vi "红绿灯.vi"() -> ()   [LabVIEW 2020]
panel:
  in  "布尔":bool caption="白天/黑夜模式"
  out "簇 十位  2":T1
  out "簇 个位 2":T1
  out "簇 十位":T1
  out "簇 个位":T1
  in  "停止":bool
  out "Elapsed Time (s)":dbl caption="已用时间(s)"
  out "南北绿[5]":bool
  out "南北黄[4]":bool
  out "南北红[3]":bool
  out "东西绿[2]":bool
  out "东西黄[1]":bool
  out "东西红[0]":bool
  # "北"
  # "西"
  # "东"
  # "南"
  # "白天"
  # "黑夜"
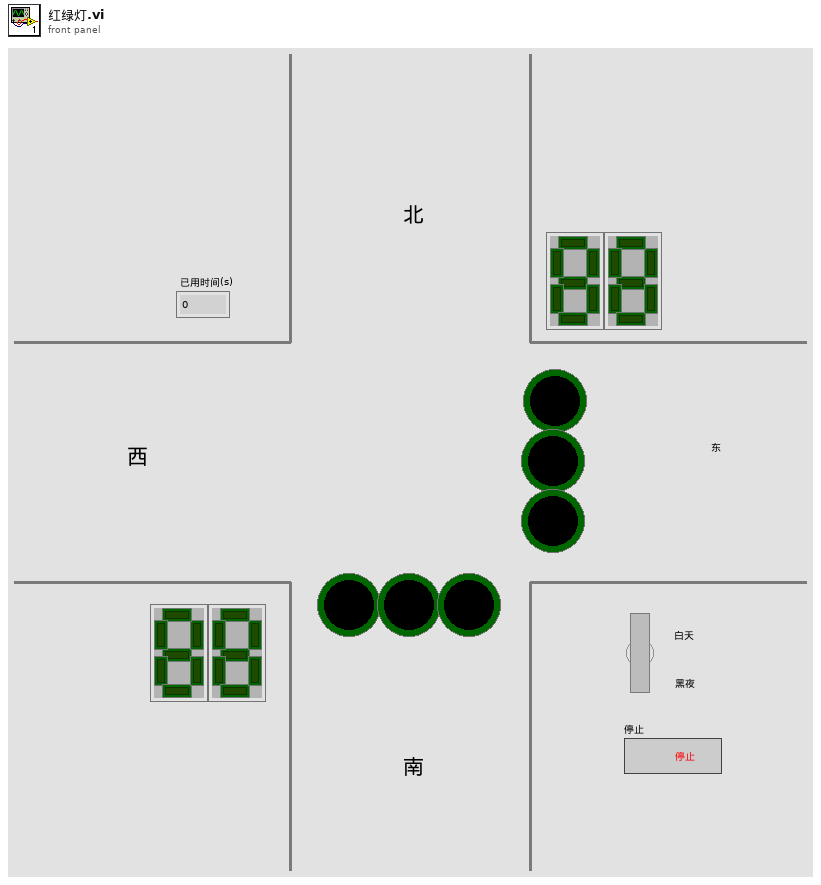
[diagram p1: front panel]
types:
  T1 = cluster{"布尔":bool, "布尔 2":bool, "布尔 3":bool, "布尔 4":bool, "布尔 5":bool, "布尔 6":bool, "布尔 7":bool}
  T2 = cluster{"布尔[0]":bool, "布尔[1]":bool, "布尔[2]":bool, "布尔[3]":bool, "布尔[4]":bool, "布尔[5]":bool}
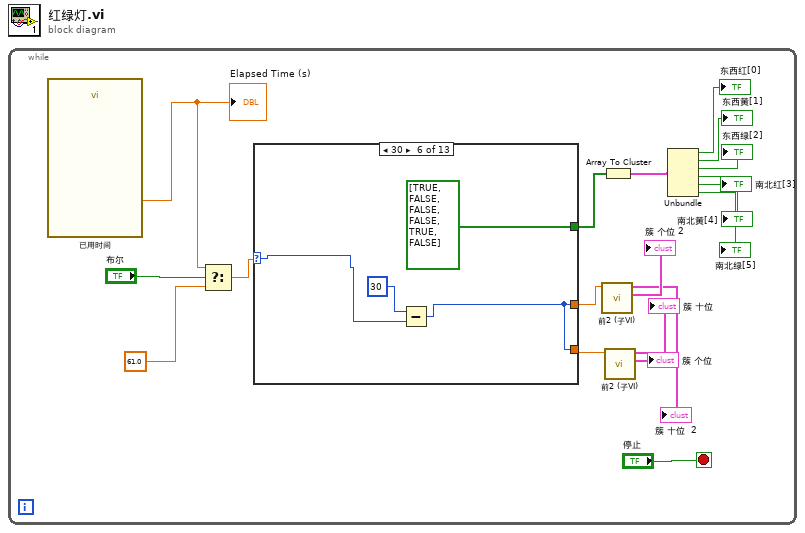
[diagram p0: block diagram]
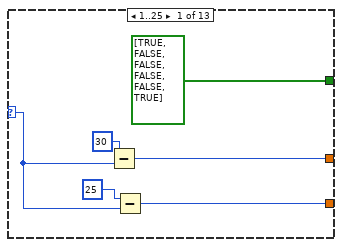
[diagram p2: hidden frame]
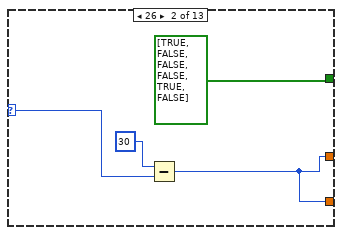
[diagram p3: hidden frame]
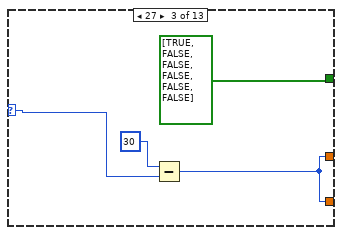
[diagram p4: hidden frame]
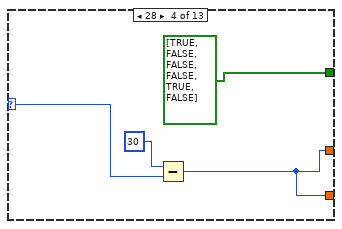
[diagram p5: hidden frame]
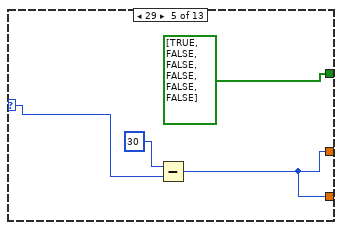
[diagram p6: hidden frame]
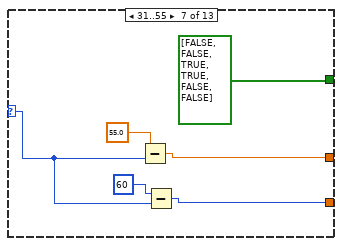
[diagram p7: hidden frame]
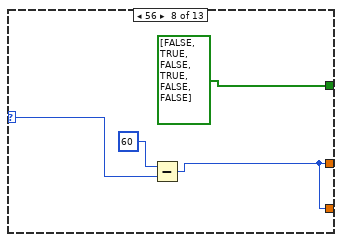
[diagram p8: hidden frame]
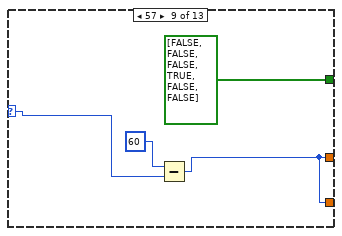
[diagram p9: hidden frame]
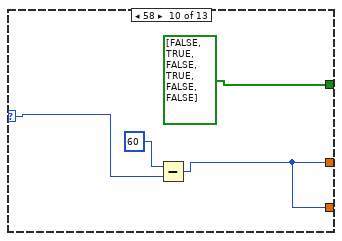
[diagram p10: hidden frame]
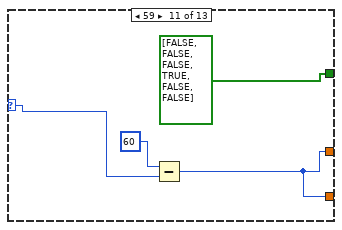
[diagram p11: hidden frame]
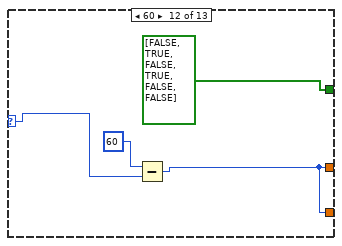
[diagram p12: hidden frame]
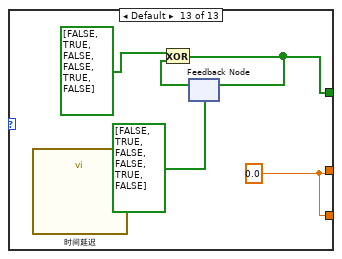
[diagram p13: hidden frame]
diagram:
  n1 = while {
    stop <- "停止" stop-if-true
    n2 = call "已用时间"() -> ("Elapsed Time (s)"=w11:dbl)  [unwired: 12 in, 7 out]
    "Elapsed Time (s)" <- w11
    n3 = Select(t=w11, s="布尔", f=61.0) -> (s? t:f=w8:dbl)
    n4 = case shown="30" w8 {
      selector: w8 -> [w20 w27 w32 w35 w39 w43 w48 w53 w57 w61 w65 w69 _]
      tunnel: [bool[] [TRUE, FALSE, FALSE, FALSE, FALSE, TRUE] ("布尔") bool[] [TRUE, FALSE, FALSE, FALSE, TRUE, FALSE] ("布尔") bool[] [TRUE, FALSE, FALSE, FALSE, FALSE, FALSE] ("布尔") bool[] [TRUE, FALSE, FALSE, FALSE, TRUE, FALSE] ("布尔") bool[] [TRUE, FALSE, FALSE, FALSE, FALSE, FALSE] ("布尔") bool[] [TRUE, FALSE, FALSE, FALSE, TRUE, FALSE] ("布尔") bool[] [FALSE, FALSE, TRUE, TRUE, FALSE, FALSE] ("布尔") bool[] [FALSE, TRUE, FALSE, TRUE, FALSE, FALSE] ("布尔") bool[] [FALSE, FALSE, FALSE, TRUE, FALSE, FALSE] ("布尔") bool[] [FALSE, TRUE, FALSE, TRUE, FALSE, FALSE] ("布尔") bool[] [FALSE, FALSE, FALSE, TRUE, FALSE, FALSE] ("布尔") bool[] [FALSE, TRUE, FALSE, TRUE, FALSE, FALSE] ("布尔") w75] -> w19
      tunnel: [w24 w26 w31 w34 w38 w42 w47 w52 w56 w60 w64 w68 w72] -> w6
      tunnel: [w23 w26 w31 w34 w38 w42 w46 w52 w56 w60 w64 w68 w72] -> w5
      frame 1..25 {
        n5 = Subtract(x=30, y=w20) -> (x-y=w24:i32)
        n6 = Subtract(x=25, y=w20) -> (x-y=w23:i32)
      }
      frame 26 {
        n7 = Subtract(x=30, y=w27) -> (x-y=w26:i32)
      }
      frame 27 {
        n8 = Subtract(x=30, y=w32) -> (x-y=w31:i32)
      }
      frame 28 {
        n9 = Subtract(x=30, y=w35) -> (x-y=w34:i32)
      }
      frame 29 {
        n10 = Subtract(x=30, y=w39) -> (x-y=w38:i32)
      }
      frame 30 {
        n11 = Subtract(x=30, y=w43) -> (x-y=w42:i32)
      }
      frame 31..55 {
        n12 = Subtract(x=55.0, y=w48) -> (x-y=w47:dbl)
        n13 = Subtract(x=60, y=w48) -> (x-y=w46:i32)
      }
      frame 56 {
        n14 = Subtract(x=60, y=w53) -> (x-y=w52:i32)
      }
      frame 57 {
        n15 = Subtract(x=60, y=w57) -> (x-y=w56:i32)
      }
      frame 58 {
        n16 = Subtract(x=60, y=w61) -> (x-y=w60:i32)
      }
      frame 59 {
        n17 = Subtract(x=60, y=w65) -> (x-y=w64:i32)
      }
      frame 60 {
        n18 = Subtract(x=60, y=w69) -> (x-y=w68:i32)
      }
      frame Default {
        w72 = 0.0 ("f")
        n19 = call "时间延迟"() -> ()  [unwired: 11 in, 1 out]
        n20 = feedback #1(bool[] [FALSE, TRUE, FALSE, FALSE, TRUE, FALSE] ("布尔")) -> (w74:bool[])
        n21 = Exclusive Or(1:w74, 2:bool[] [FALSE, TRUE, FALSE, FALSE, TRUE, FALSE] ("布尔")) -> (0:w75:bool[])
        n22 = feedback-in #1(w75) -> ()
      }
    }
    n23 = call "前2 (子VI).vi"("x"=w6) -> ("簇 个位"=→"簇 个位 2":T1, "簇 十位"=→"簇 十位  2":T1)  [unwired: 8 in]
    n24 = Array To Cluster(array=w19) -> (cluster=w18:T2)
    n25 = call "前2 (子VI).vi"("x"=w5) -> ("簇 个位"=→"簇 个位":T1, "簇 十位"=→"簇 十位":T1)  [unwired: 8 in]
    n26 = Unbundle(w18) -> ("布尔[0]"=→"东西红[0]":bool, "布尔[1]"=→"东西黄[1]":bool, "布尔[2]"=→"东西绿[2]":bool, "布尔[3]"=→"南北红[3]":bool, "布尔[4]"=→"南北黄[4]":bool, "布尔[5]"=→"南北绿[5]":bool)
  }
